vi "_Read Users From File.vi"(8 "Error in":errorcluster caption="Error in (no error)") -> (0 "Error out":errorcluster, 3 "Array":T1[](array[typedef]))   [LabVIEW 2017, in "Login-UI.lvlib"]
uses:
  Login-UI.lvlib
  _Typedef/User-Info.ctl
  _Typedef/User-Role.ctl
  0a74098a-8fda-4e50-8bcc-1f710fccc8a0.vi
  0eb53b96-9a7b-45e4-8871-4f0d25c26834.vi
  <userlib>/NEVSTOP-Programming-Palette/Configuration/ClusterCfgTable/Parse CfgTable(with DataName).vi
  <userlib>/NEVSTOP-Programming-Palette/Configuration/Ini/ini_configuration_nevstop.lvlib
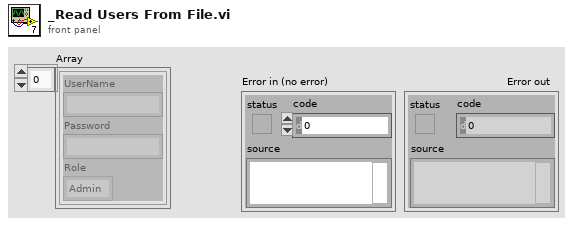
[diagram p1: front panel]
types:
  T1 = typedef "Login-UI.lvlib/User-Info.ctl" = cluster{"UserName":string, "Password":string, "Role":T2}
  T2 = typedef "Login-UI.lvlib/User-Role.ctl" = enum16{"INVALID", "Operator", "Engineer", "Admin"}
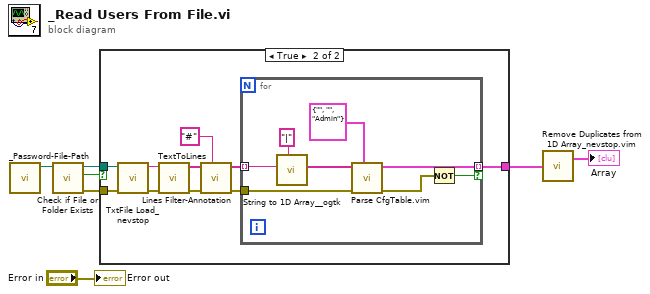
[diagram p0: block diagram]
diagram:
  n1 = call "_Password-File-Path.vi"() -> ("Matched Config File"=w3:path)  [unwired: 11 in]
  n2 = call <vilib>:"Check if File or Folder Exists.vi"("path"=w3) -> ("error out"=w5:errorcluster, "file or folder exists?"=w6:bool, "dup path"=w4:path)  [unwired: 8 in]
  n3 = case shown="True" w6 {
    tunnel: w4 -> [_ w11]
    tunnel: w5 -> [_ w10]
    tunnel: [_ w9] -> w7
    frame False {
    }
    frame True {
      n4 = call <userlib>:"TxtFile Load_nevstop.vi"("error in (no error)"=w10, "Path"=w11) -> ("error out"=w17:errorcluster, "text"=w16:string)  [unwired: 8 in]
      n5 = call <userlib>:"TextToLines.vi"("error in (no error)"=w17, "string"=w16) -> ("error out"=w15:errorcluster, "Lines"=w14:string[])  [unwired: 8 in]
      n6 = call <userlib>:"Lines Filter-Annotation.vi"("Annotation Seperator(#)"="#", "error in (no error)"=w15, "Lines"=w14) -> ("error out"=w12:errorcluster, "Config Text List"=w13:string[])  [unwired: 7 in]
      n7 = for {
        tunnel: w13 -> [w25] mode=indexing
        tunnel: w12 -> [w24]
        tunnel: [w20] -> w9 mode=indexing if=w18
        n8 = call <userlib>:"String to 1D Array__ogtk.vi"("delimiter (Tab)"="|", "string"=w25) -> ("Array of Strings"=w23:string[])  [unwired: 9 in]
        n9 = call "Parse CfgTable.vim"("Cluster Configuration Typedef"=T1 {"UserName"="", "Password"="", "Role"=enum."Admin"}, "error in (no error)"=w24, "CfgTable Row"=w23) -> ("error out"=w19:errorcluster, "Cluster Configuration Out"=w20:T1)  [unwired: 7 in]
        n10 = Not(x=w19) -> (.not. x?=w18:bool)
      }
    }
  }
  n11 = call "Remove Duplicates from 1D Array_nevstop.vim"("Input Array"=w7) -> ("Output Array"=→"Array":T1[])  [unwired: 1 out]
  "Error out" <- "Error in"
